vi "Read String in C.vi"(8 "error in (no error)":errorcluster, 11 "C in":refnum<class "C.lvclass">) -> (0 "error out":errorcluster, 2 "String in C":string, 3 "C out":refnum<class "C.lvclass">)   [LabVIEW 2013, in "C.lvclass"]
uses:
  C.lvclass
  C.lvclass/C.ctl
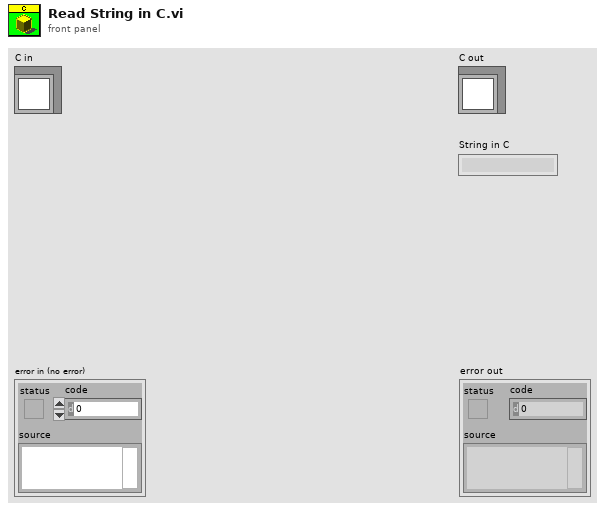
[diagram p1: front panel]
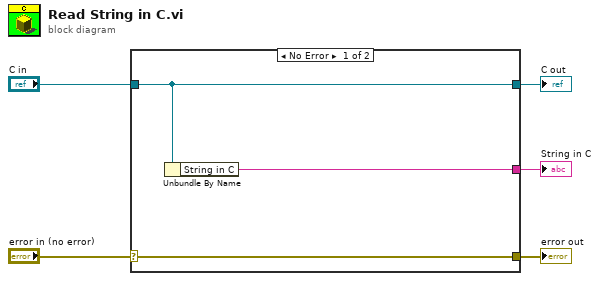
[diagram p0: block diagram]
diagram:
  n1 = case shown="No Error" "error in (no error)" {
    selector: "error in (no error)" -> [w8 w9]
    tunnel: [w8 w9] -> w4
    tunnel: [w7 w10] -> w2
    tunnel: "C in" -> [w7 w10]
    tunnel: [w6 _] -> w1
    frame No Error {
      n2 = Unbundle By Name(w7) -> ("String in C"=w6:string)
    }
    frame Error {
    }
  }
  "error out" <- w4
  "C out" <- w2
  "String in C" <- w1
